vi "string_to_log_event.vi"(0 "String":string, 11 "error in":errorcluster) -> (4 "Log event":T1 {"Timestamp" format="%<%.3X>T"}, 15 "error out":errorcluster)   [LabVIEW 2012]
uses:
  log_event.ctl
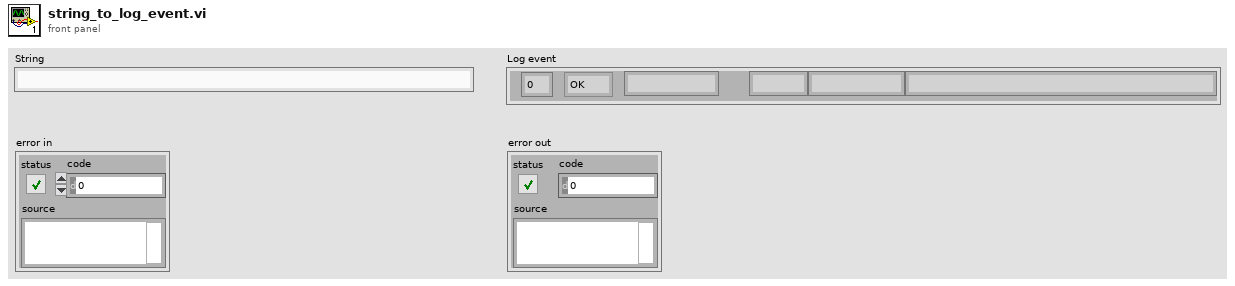
[diagram p1: front panel]
types:
  T1 = typedef "log_event.ctl" = cluster{"Facility ID":i32, "Severity":enum16{"OK", "Debug", "Warn", "Error"}, "Timestamp":timestamp, "Facility":string, "State":string, "Message":string}
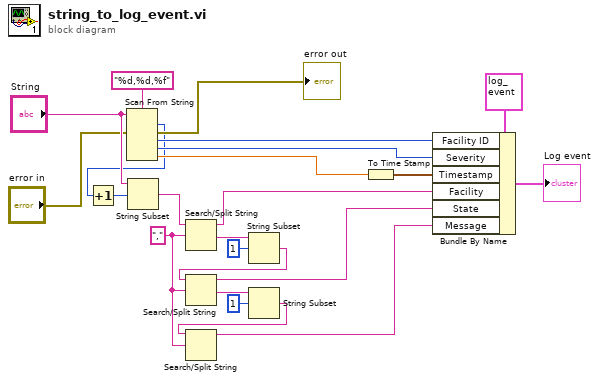
[diagram p0: block diagram]
diagram:
  w8 = "," ("search string/char (-)")
  n1 = Scan From String(format string="%d,%d,%f", input string="String", error in="error in") -> (offset past scan=w3:u32, error out=→"error out":errorcluster, output 1=w21:i32, output 2=w20:i32, output 3=w19:dbl)  [unwired: 4 in, 1 out]
  n2 = Increment(x=w3) -> (x+1=w2:u32)
  n3 = String Subset(string="String", offset (0)=w2) -> (substring=w4:string)  [unwired: 1 in]
  n4 = Search/Split String(string=w4, search string/char (-)=w8) -> (substring before match=w15:string, match + rest of string=w14:string)  [unwired: 1 in, 1 out]
  n5 = String Subset(string=w14, offset (0)=1) -> (substring=w10:string)  [unwired: 1 in]
  n6 = Search/Split String(string=w10, search string/char (-)=w8) -> (substring before match=w7:string, match + rest of string=w11:string)  [unwired: 1 in, 1 out]
  n7 = String Subset(string=w11, offset (0)=1) -> (substring=w9:string)  [unwired: 1 in]
  n8 = Search/Split String(string=w9, search string/char (-)=w8) -> (substring before match=w6:string)  [unwired: 1 in, 2 out]
  n9 = To Time Stamp(1:w19) -> (0:w18:timestamp)
  n10 = Bundle By Name(cluster=T1 {"Facility ID"=0, "Severity"=enum."OK", "Timestamp"=timestamp(0 s since 1904-01-01), "Facility"="", "State"="", "Message"=""} ("Log event"), "Facility ID"=w21, "Severity"=w20, "Timestamp"=w18, "Facility"=w15, "State"=w7, "Message"=w6) -> (→"Log event":T1)
